vi "DataLog.vi"(1 "array":dbl[](array[numeric])) -> (0 "Result":string)   [LabVIEW 2021]
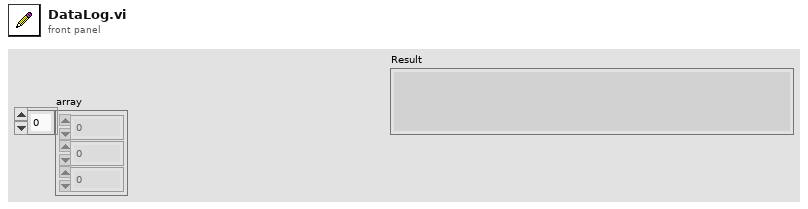
[diagram p1: front panel]
types:
  T1 = cluster{"array[0]":dbl, "array[1]":dbl, "array[2]":dbl, "array[3]":dbl, "array[4]":dbl, "array[5]":dbl, "array[6]":dbl, "array[7]":dbl, "array[8]":dbl}
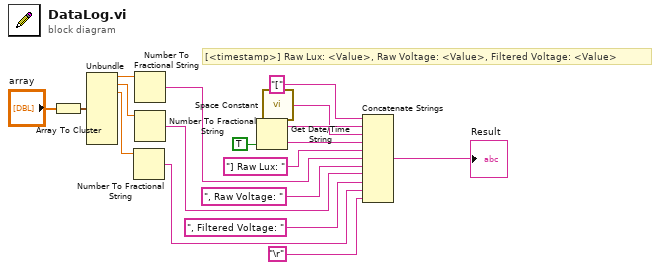
[diagram p0: block diagram]
diagram:
  # "[<timestamp>] Raw Lux: <Value>, Raw Voltage: <Value>, Filtered Voltage: <Value>"
  n1 = Array To Cluster(array="array") -> (cluster=w7:T1)
  n2 = Unbundle(w7) -> ("array[0]"=w6:dbl, "array[1]"=w2:dbl, "array[2]"=w1:dbl)  [unwired: 6 out]
  n3 = Number To Fractional String(number=w1) -> (F-format string=w3:string)  [unwired: 3 in]
  n4 = Number To Fractional String(number=w6) -> (F-format string=w5:string)  [unwired: 3 in]
  n5 = Number To Fractional String(number=w2) -> (F-format string=w4:string)  [unwired: 3 in]
  n6 = Get Date/Time String(want seconds? (F)=TRUE) -> (date string=w16:string, time string=w15:string)  [unwired: 2 in]
  n7 = call <vilib>:"Space Constant.vi"() -> ("String"=w14:string)
  n8 = Concatenate Strings("[" ("string"), w16, w14, w15, "] Raw Lux: " ("string"), w5, ", Raw Voltage: " ("string"), w4, ", Filtered Voltage: " ("string"), w3, "\r") -> (→"Result":string)
